vi "Simulated Temperature Chamber Example.vi"() -> ()   [LabVIEW 2020]
uses:
  <vilib>/Skyline/Tag/Shared/typedefs/DataType.ctl
  <vilib>/Skyline/Tag/Wrapper/Wrapper AMQP_class/Open Tag AMQP.vi
  <vilib>/Skyline/Tag/Wrapper/Wrapper_class/Write Tag (DBL).vi
  <vilib>/Skyline/Tag/Wrapper/Wrapper_class/Close Tag (Single).vi
  FlexLoggerTagHelpers.lvlib
  <vilib>/Skyline/Tag/Wrapper/Wrapper_class/NI Skyline Tag.lvclass
  <vilib>/Skyline/Tag/Wrapper/Wrapper AMQP_class/NI Skyline Tag AMQP.lvclass
  <vilib>/Skyline/Tag/Shared/NI Skyline Tag.lvlib
panel:
  out "Chamber Temperatures":T1(graph)
  in  "Stop":bool
  # "Overview: This example shows how to plug in external data to FlexLogger using SystemLink Tags.  Simulated temperature\nreadings from a chamber are written to FlexLogger SystemLink tags at a rate ten updates per second.\nRequirements: LabVIEW Full Development System, FlexLogger\nInstructions:\n1. Launch FlexLogger\n     a. Create a Project.\n     b. Using the Project >> Settings menu, enable Publish SystemLink Tags (Export) and Consume External SystemLink Tags (Import).\n     c. Restart the FlexLogger Project.\n2. Run this VI. \n3. Within the FlexLogger project:\n     a. Note that the new exported tags appear in the Channel Specification page.\n     b. Switch to the Screen document, drop a Long History Graph, and connect the new tag channels to the graph.\n4. Click on the Stop button to stop this VI and close all SystemLink tags.  \n5. Note that in FlexLogger all channels connected to the temperature tags will no longer update."
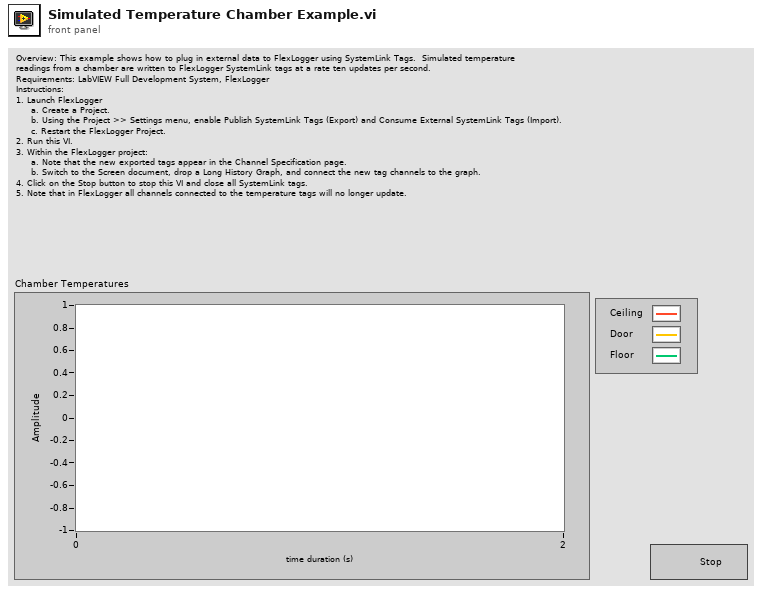
[diagram p1: front panel]
types:
  T1 = cluster{"Floor Temperature":dbl, "Ceiling Temperature":dbl, "Door Temperature":dbl}
  T2 = typedef "NI Skyline Tag.lvlib/DataType.ctl" = enum32{"Double", "I32", "String", "Boolean", "U64", "Timestamp"}
  T3 = cluster{"Ceiling Temperature":dbl, "Door Temperature":dbl, "Floor Temperature":dbl}
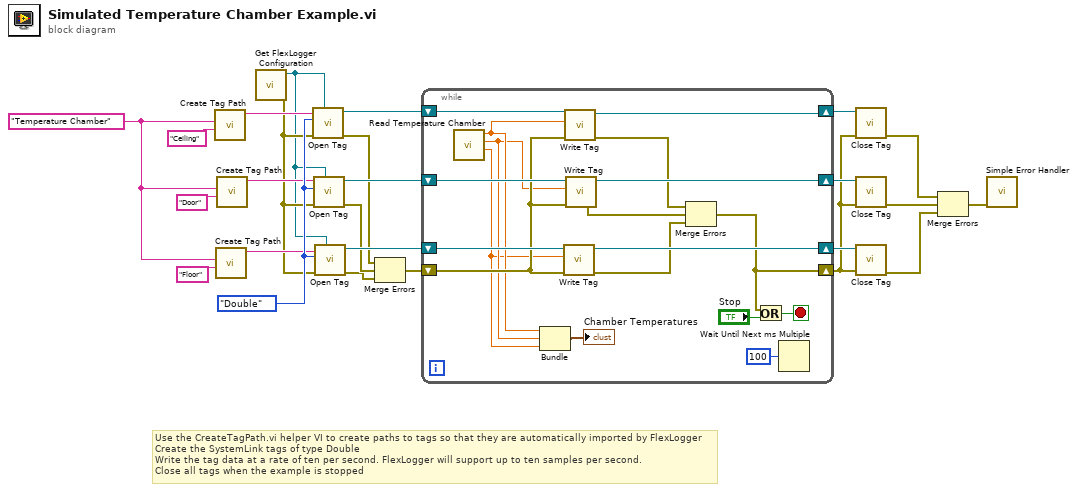
[diagram p0: block diagram]
diagram:
  w22 = "Temperature Chamber" ("Group Name")
  w25 = DataType."Double" ("data type")
  # "Use the CreateTagPath.vi helper VI to create paths to tags so that they are automatically imported by FlexLogger\nCreate the SystemLink tags of type Double\nWrite the tag data at a rate of ten per second. FlexLogger will support up to ten samples per second.\nClose all tags when the example is stopped"
  n1 = call "Create Tag Path.vi"("channel name"="Ceiling" ("Channel Name"), "group name"=w22) -> ("tag path"=w23:string)  [unwired: 9 in]
  n2 = call "Create Tag Path.vi"("channel name"="Floor" ("Channel Name"), "group name"=w22) -> ("tag path"=w18:string)  [unwired: 9 in]
  n3 = call "Create Tag Path.vi"("channel name"="Door" ("Channel Name"), "group name"=w22) -> ("tag path"=w24:string)  [unwired: 9 in]
  n4 = call "Get FlexLogger Configuration.vi"() -> ("error out"=w2:errorcluster, "Local FlexLogger Configuration"=w1:refnum<class "NI Skyline Configuration AMQP.lvclass">)  [unwired: 10 in]
  n5 = call-poly <vilib>:"Open Tag.vi"("configuration"=w1, "error in (no error)"=w2, "data type"=w25, "path"=w23) -> ("error out"=w14:errorcluster, "tag"=w16:refnum<class "NI Skyline Tag.lvclass">)  [unwired: 6 in]
  n6 = call-poly <vilib>:"Open Tag.vi"("configuration"=w1, "error in (no error)"=w2, "data type"=w25, "path"=w24) -> ("error out"=w13:errorcluster, "tag"=w15:refnum<class "NI Skyline Tag.lvclass">)  [unwired: 6 in]
  n7 = call-poly <vilib>:"Open Tag.vi"("configuration"=w1, "error in (no error)"=w2, "data type"=w25, "path"=w18) -> ("error out"=w12:errorcluster, "tag"=w17:refnum<class "NI Skyline Tag.lvclass">)  [unwired: 6 in]
  n8 = Merge Errors(w14, w13, w12) -> (w11:errorcluster)
  n9 = while {
    shift-right: [w37] -> w9
    shift-left: w15 -> [w43]
    shift-right: [w36] -> w8
    shift-left: w16 -> [w39]
    shift-right: [w35] -> w10
    shift-left: w17 -> [w40]
    shift-right: [w31] -> w7
    shift-left: w11 -> [w30]
    stop <- w41 stop-if-true
    n10 = call "Read Temperature Chamber.vi"() -> ("Floor Temperature"=w27:dbl, "Door Temperature"=w28:dbl, "Ceiling Temperature"=w29:dbl)  [unwired: 9 in]
    n11 = Bundle("Ceiling Temperature"=w29, "Door Temperature"=w28, "Floor Temperature"=w27) -> (→"Chamber Temperatures":T3)  [unwired: 1 in]
    n12 = call-poly <vilib>:"Write Tag.vi"("error in (no error)"=w30, "value"=w27, "tag in"=w40) -> ("error out"=w32:errorcluster, "tag out"=w35:refnum<class "NI Skyline Tag.lvclass">)  [unwired: 7 in]
    n13 = call-poly <vilib>:"Write Tag.vi"("error in (no error)"=w30, "value"=w29, "tag in"=w39) -> ("error out"=w34:errorcluster, "tag out"=w36:refnum<class "NI Skyline Tag.lvclass">)  [unwired: 7 in]
    n14 = call-poly <vilib>:"Write Tag.vi"("error in (no error)"=w30, "value"=w28, "tag in"=w43) -> ("error out"=w33:errorcluster, "tag out"=w37:refnum<class "NI Skyline Tag.lvclass">)  [unwired: 7 in]
    n15 = Merge Errors(w34, w33, w32) -> (w31:errorcluster)
    n16 = Or(x=w31, y="Stop") -> (x .or. y?=w41:bool)
    n17 = Wait Until Next ms Multiple(millisecond multiple=u32 100 ("milliseconds to wait")) -> ()  [unwired: 1 out]
  }
  n18 = call-poly <vilib>:"Close Tag.vi"("error in (no error)"=w7, "tag"=w8) -> ("error out"=w6:errorcluster)  [unwired: 9 in]
  n19 = call-poly <vilib>:"Close Tag.vi"("error in (no error)"=w7, "tag"=w9) -> ("error out"=w5:errorcluster)  [unwired: 9 in]
  n20 = call-poly <vilib>:"Close Tag.vi"("error in (no error)"=w7, "tag"=w10) -> ("error out"=w4:errorcluster)  [unwired: 9 in]
  n21 = Merge Errors(w6, w5, w4) -> (w3:errorcluster)
  n22 = call <vilib>:"Simple Error Handler.vi"("error in (no error)"=w3) -> ()  [unwired: 4 in, 5 out]
